vi "Create Object.vi"(11 "Dev Panel in":refnum<class "Dev Panel.lvclass">) -> (3 "Dev Panel out":refnum<class "Dev Panel.lvclass">)   [LabVIEW 2021, in "Dev Panel.lvclass"]
uses:
  Dev Panel.lvclass
  Dev Panel.lvclass/Dev Panel.ctl
  jettl/jettl.lvlib
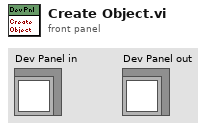
[diagram p1: front panel]
types:
  T1 = cluster{"Events":cluster{"Teardown":refnum<user-event>, "Pop Up":refnum<user-event>, "String Indicator":refnum<user-event>, "Button":refnum<user-event>}, "Refs":cluster{"FP Ref":refnum<vi>, "Pop Up":refnum<vi>, "String Indicator":refnum<vi>, "Button":refnum<vi>}, "BG Color":u32, "Event Actor":refnum<class "Event Actor.lvclass">}
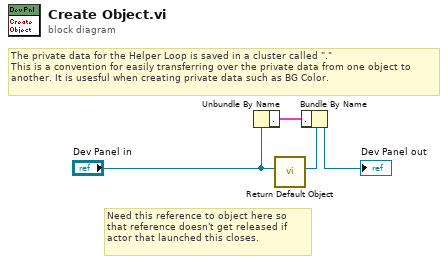
[diagram p0: block diagram]
diagram:
  # "The private data for the Helper Loop is saved in a cluster called \".\"\nThis is a convention for easily transferring over the private data from one object to another. It is usesful when creating private data such as BG Color."
  # "Need this reference to object here so that reference doesn't get released if actor that launched this closes."
  n1 = Unbundle By Name("Dev Panel in") -> ("."=w4:T1)
  n2 = call "Return Default Object.vi"("Object"="Dev Panel in") -> ("Default Object Instance"=w2:refnum<class "Dev Panel.lvclass">)  [unwired: 10 in]
  n3 = Bundle By Name(cluster=w2, "."=w4) -> (→"Dev Panel out":refnum<class "Dev Panel.lvclass">)
